vi "Node - PXImc Connect.vi"(8 "error in (no error)":errorcluster, 11 "Node Data In in":T1) -> (0 "error out":errorcluster, 3 "Node Data In out":T1)   [LabVIEW 2016, in "PXImc Router.lvlib"]
uses:
  PXImc Router.lvlib
  Controls/Node/Node - Config.ctl
  <vilib>/NI Veristand/VeriStand Data/Byte Buffer/Byte Buffer.lvclass
  Controls/Node/Node - PXImc Parameters.ctl
  Controls/Node/Node - Writer Data.ctl
  Controls/Node/Node - Ch Properties.ctl
  Controls/Data Type.ctl
  Controls/Node/Node - Readers Data.ctl
  Controls/Node/Node - Reader Data.ctl
  <vilib>/pximc/Connect (U8).vi
  <vilib>/pximc/nipximc.lvlib
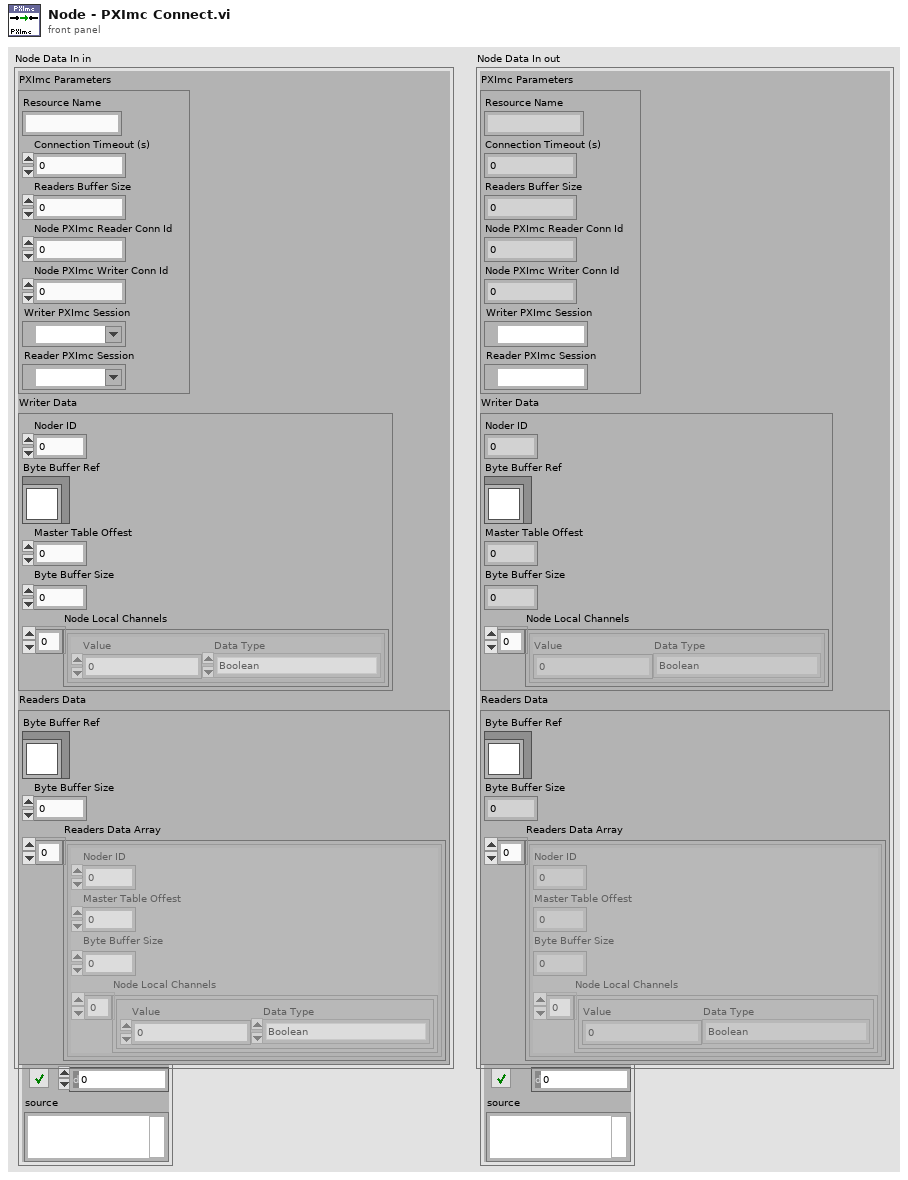
[diagram p1: front panel]
types:
  T1 = typedef "PXImc Router.lvlib/Node - Config.ctl" = cluster{"PXImc Parameters":T2, "Writer Data":T3, "Readers Data":T6}
  T2 = typedef "PXImc Router.lvlib/Node - PXImc Parameters.ctl" = cluster{"Resource Name":string, "Connection Timeout (s)":dbl, "Readers Buffer Size":u64, "Node PXImc Reader Conn Id":u16, "Node PXImc Writer Conn Id":u16, "Writer PXImc Session":refnum<k21>, "Reader PXImc Session":refnum<k21>}
  T3 = typedef "PXImc Router.lvlib/Node - Writer Data.ctl" = cluster{"Noder ID":u32, "Byte Buffer Ref":refnum<class "Byte Buffer.lvclass">, "Master Table Offest":u32, "Byte Buffer Size":u32, "Node Local Channels":T4[]}
  T4 = typedef "PXImc Router.lvlib/Node - Ch Properties.ctl" = cluster{"Value":dbl, "Data Type":T5}
  T5 = typedef "PXImc Router.lvlib/Data Type.ctl" = enum16{"Boolean", "SGL", "DBL", "I8", "I16", "I32", "I64", "U8", "U16", "U32", "U64"}
  T6 = typedef "PXImc Router.lvlib/Node - Readers Data.ctl" = cluster{"Byte Buffer Ref":refnum<class "Byte Buffer.lvclass">, "Byte Buffer Size":u64, "Readers Data Array":T7[]}
  T7 = typedef "PXImc Router.lvlib/Node - Reader Data.ctl" = cluster{"Noder ID":u32, "Master Table Offest":u32, "Byte Buffer Size":u64, "Node Local Channels":T4[]}
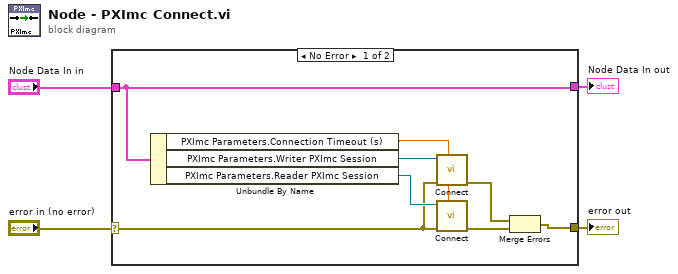
[diagram p0: block diagram]
diagram:
  n1 = case shown="No Error" "error in (no error)" {
    selector: "error in (no error)" -> [w10 w13]
    tunnel: "Node Data In in" -> [w5 w14]
    tunnel: [w5 w14] -> w2
    tunnel: [w7 w13] -> w4
    frame No Error {
      n2 = Unbundle By Name(w5) -> ("PXImc Parameters.Connection Timeout (s)"=w6:dbl, "PXImc Parameters.Writer PXImc Session"=w11:refnum<k21>, "PXImc Parameters.Reader PXImc Session"=w12:refnum<k21>)
      n3 = call-poly <vilib>:"Connect.vi"("timeout in seconds (-1)"=w6, "error in (no error)"=w10, "session in"=w11) -> ("error out"=w9:errorcluster)  [unwired: 7 in, 1 out]
      n4 = call-poly <vilib>:"Connect.vi"("timeout in seconds (-1)"=w6, "error in (no error)"=w10, "session in"=w12) -> ("error out"=w8:errorcluster)  [unwired: 7 in, 1 out]
      n5 = Merge Errors(w9, w8) -> (w7:errorcluster)
    }
    frame Error {
    }
  }
  "error out" <- w4
  "Node Data In out" <- w2
